vi "init.vi"(8 "error in (no error)":errorcluster, 11 "Model in":refnum<class "Model.lvclass">) -> (0 "error out":errorcluster, 3 "Model out":refnum<class "Model.lvclass">)   [LabVIEW 2016, in "Model.lvclass"]
doc: "Reads the configuration and prepares the PubDataSVs."
uses:
  Model.lvclass
  Model.lvclass/Model.ctl
  Target/Target/Target.lvclass
  ComponentTemplateCore/ComponentModel/ComponentModelRT/LoopTimer/ILoopTimer/ILoopTimer.lvclass
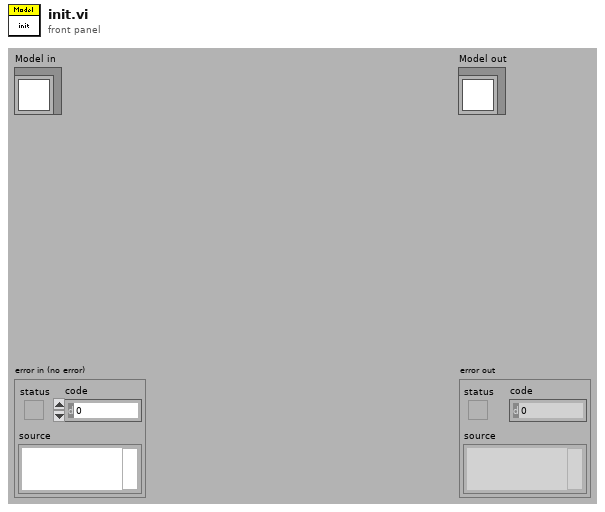
[diagram p1: front panel]
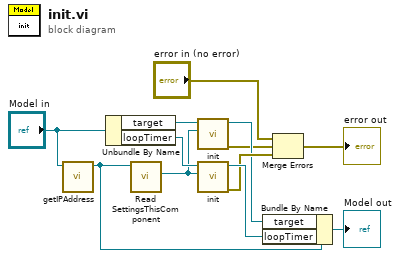
[diagram p0: block diagram]
diagram:
  n1 = call-dynamic "getIPAddress.vi"("Model in"="Model in") -> ("Model out"=w1:refnum<class "Model.lvclass">)  [unwired: 9 in, 1 out]
  n2 = Unbundle By Name("Model in") -> ("target"=w5:refnum<class "Target.lvclass">, "loopTimer"=w12:refnum<class "ILoopTimer.lvclass">)
  n3 = call-dynamic "Read SettingsThisComponent.vi"("Model in"=w1) -> ("Settings.lvlib:TCSettings.lvclass"=w3:refnum<class "TCSettings.lvclass">)  [unwired: 8 in, 2 out]
  n4 = call-dynamic "init.vi"("Settings.lvlib:TCSettings.lvclass"=w3, "Target in"=w5) -> ("error out"=w6:errorcluster, "Target out"=w7:refnum<class "Target.lvclass">)  [unwired: 8 in]
  n5 = call-dynamic "init.vi"("Settings.lvlib:TCSettings.lvclass"=w3, "ILoopTimer in"=w12) -> ("error out"=w8:errorcluster, "ILoopTimer out"=w11:refnum<class "ILoopTimer.lvclass">)  [unwired: 8 in]
  n6 = Bundle By Name(cluster=w1, "target"=w7, "loopTimer"=w11) -> (→"Model out":refnum<class "Model.lvclass">)
  n7 = Merge Errors("error in (no error)", w6, w8) -> (→"error out":errorcluster)
